vi "Compute (Array).vi"(8 "error in (no error)":errorcluster, 10 "Data Points in":T1, 11 "Normalize in":refnum<class "Normalize.lvclass">) -> (0 "error out":errorcluster, 2 "Data Points out":T1, 3 "Normalize out":refnum<class "Normalize.lvclass">)   [LabVIEW 2009, in "Normalize.lvclass"]
doc: "Process and return an array of data points at the end of a scan. (For example, to normalize the output or find min/max, one must know all data points a priori.)"
uses:
  Normalize.lvclass
  Instruments/Utility Classes/Readable/Data Points.ctl
  Instruments/Utility Classes/Readable/Data Point.ctl
  <vilib>/Analysis/baseanly.llb/Normalize Vector.vi
  <vilib>/Analysis/NI_AALBase.lvlib
  Instruments/Utility Classes/Readable/Readable.lvclass
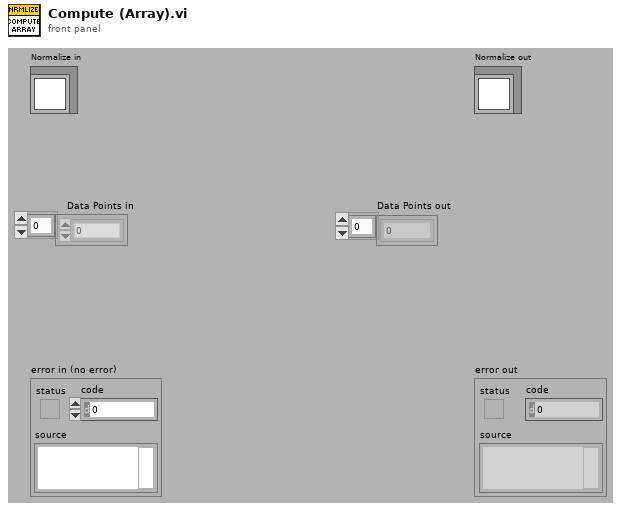
[diagram p1: front panel]
types:
  T1 = typedef "Readable.lvclass/Data Points.ctl" = T2[]
  T2 = typedef "Readable.lvclass/Data Point.ctl" = dbl
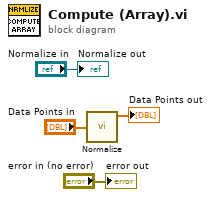
[diagram p0: block diagram]
diagram:
  n1 = call-poly <vilib>:"Normalize.vi"("Vector"="Data Points in") -> ("Normalized Vector"=→"Data Points out":dbl[])  [unwired: 1 in, 3 out]
  "error out" <- "error in (no error)"
  "Normalize out" <- "Normalize in"
